vi "Route Switch.vi"(8 "error in (no error)":errorcluster, 9 "Route to:":T1=enum."Channel 2", 10 "Route From:":T1, 11 "EXFO in":refnum<class "EXFO.lvclass">) -> (0 "error out":errorcluster, 3 "EXFO out":refnum<class "EXFO.lvclass">)   [LabVIEW 2018, in "EXFO.lvlib" / "EXFO.lvclass"]
doc: "This is a dynamically dispatched VI. The child class will set the optical signal path through the switch. EXFO switches can handle up to 16 channels. Be sure to verify if there are less than 16 channels that the input values are within the range of installed switch routes.\n\nAuthor: Ron Dexter\nCompany: Luminar\nModified: 5/20/2018"
uses:
  EXFO.lvclass
  Private/Switch Channels.ctl
  EXFO.lvlib
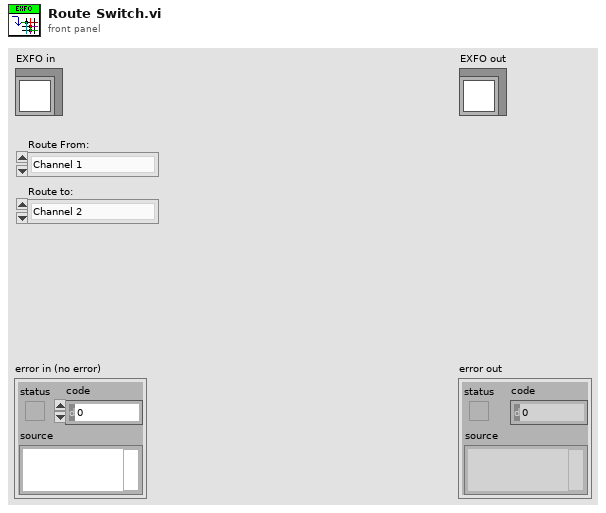
[diagram p1: front panel]
types:
  T1 = typedef "EXFO.lvlib/Switch Channels.ctl" = enum16{"Channel 1", "Channel 2", "Channel 3", "Channel 4", "Channel 5", "Channel 6", "Channel 7", "Channel 8", "Channel 9", "Channel 10", "Channel 11", "Channel 12", "Channel 13", "Channel 14", "Channel 15", "Channel 16"}
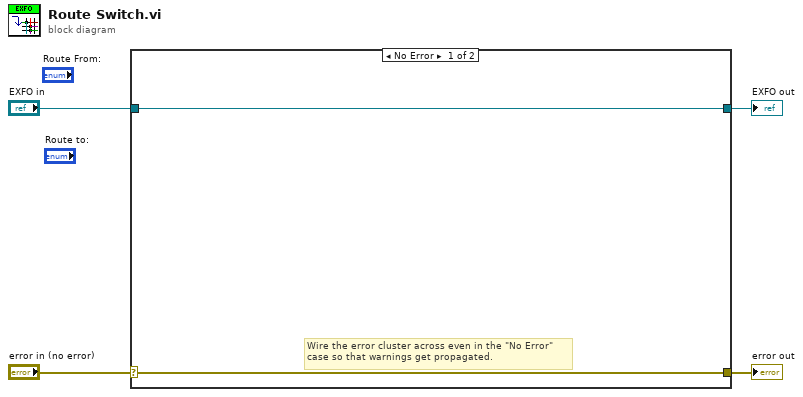
[diagram p0: block diagram]
diagram:
  n1 = case shown="No Error" "error in (no error)" {
    selector: "error in (no error)" -> [w5 w8]
    tunnel: [w5 w8] -> w3
    tunnel: [w6 w7] -> w1
    tunnel: "EXFO in" -> [w6 w7]
    frame No Error {
      # "Wire the error cluster across even in the \"No Error\"\ncase so that warnings get propagated."
    }
    frame Error {
    }
  }
  "error out" <- w3
  "EXFO out" <- w1
